vi "sumLinesIntoProjections.vi"(6 "calc ff/fb":bool, 7 "tracking":bool, 8 "error in (no error)":errorcluster, 10 "volumes to assemble":T3[](array[typedef])) -> (0 "error out":errorcluster, 1 "lines inserted":i32, 2 "volumes to send":cluster{"volume info":T1, "buffers":T2}[](array[cluster]), 3 "ch sums":cluster{"ch0 sum":u32, "ch1 sum":u32})   [LabVIEW 2010]
uses:
  volume_with_lines.ctl
  volume_info.ctl
  line_info.ctl
  projection buffers.ctl
  get write location projection.vi
  sum line into array.vi
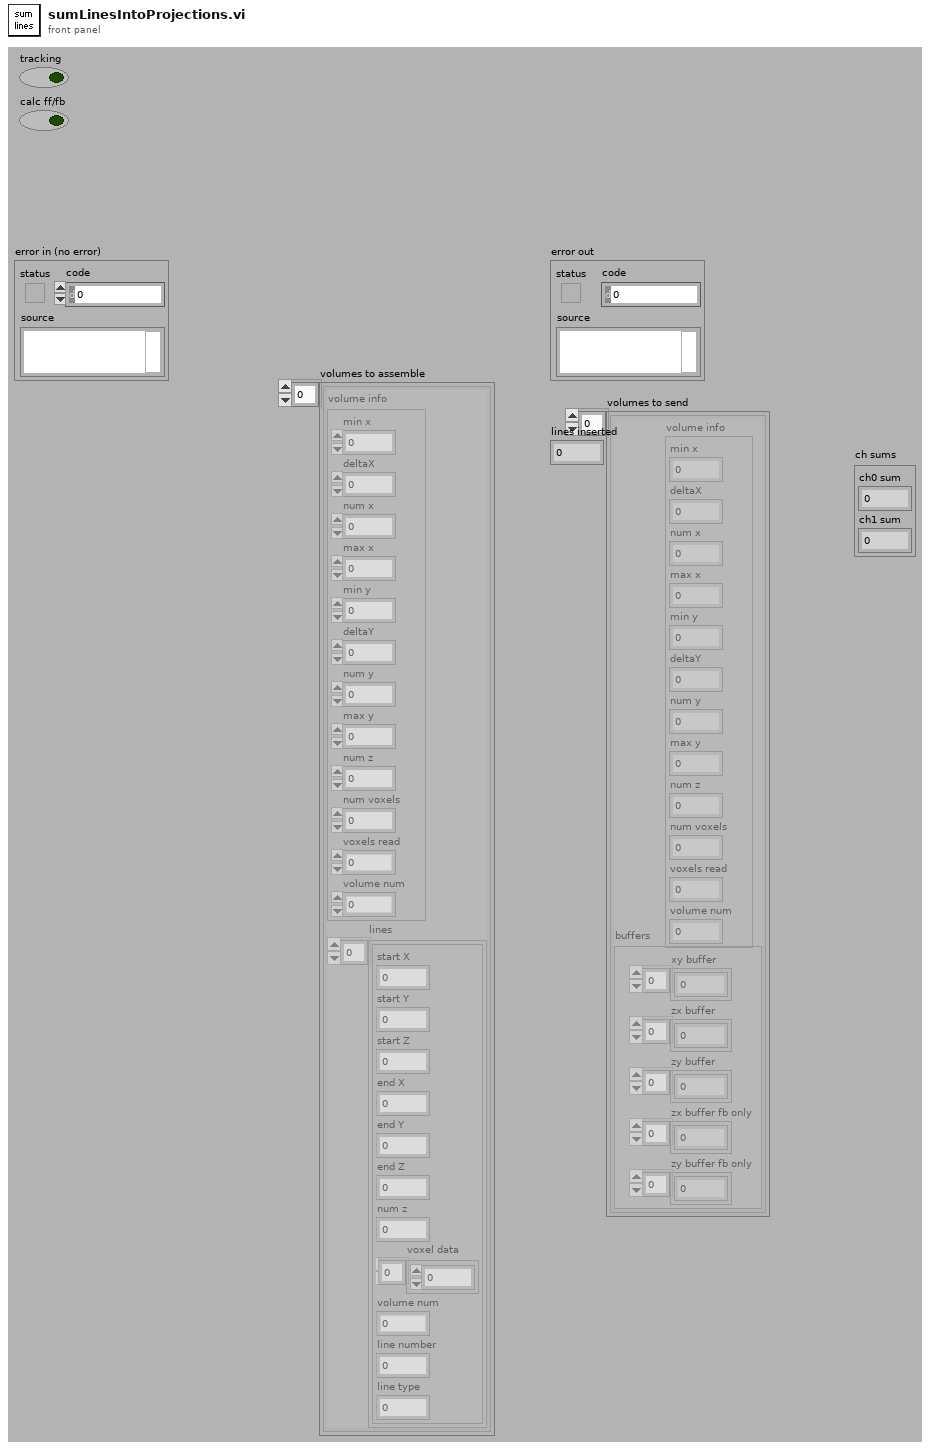
[diagram p1: front panel]
types:
  T1 = typedef "volume_info.ctl" = cluster{"min x":i16, "deltaX":dbl, "num x":u32, "max x":i16, "min y":i16, "deltaY":dbl, "num y":u32, "max y":i16, "num z":u32, "num voxels":u32, "voxels read":u32, "volume num":u32}
  T2 = typedef "projection buffers.ctl" = cluster{"xy buffer":u32[], "zx buffer":u32[], "zy buffer":u32[], "zx buffer fb only":u32[], "zy buffer fb only":u32[]}
  T3 = typedef "volume_with_lines.ctl" = cluster{"volume info":T1, "lines":T4[]}
  T4 = typedef "line_info.ctl" = cluster{"start X":i16, "start Y":i16, "start Z":i16, "end X":i16, "end Y":i16, "end Z":i16, "num z":u8, "voxel data":u32[], "volume num":u32, "line number":u16, "line type":u16}
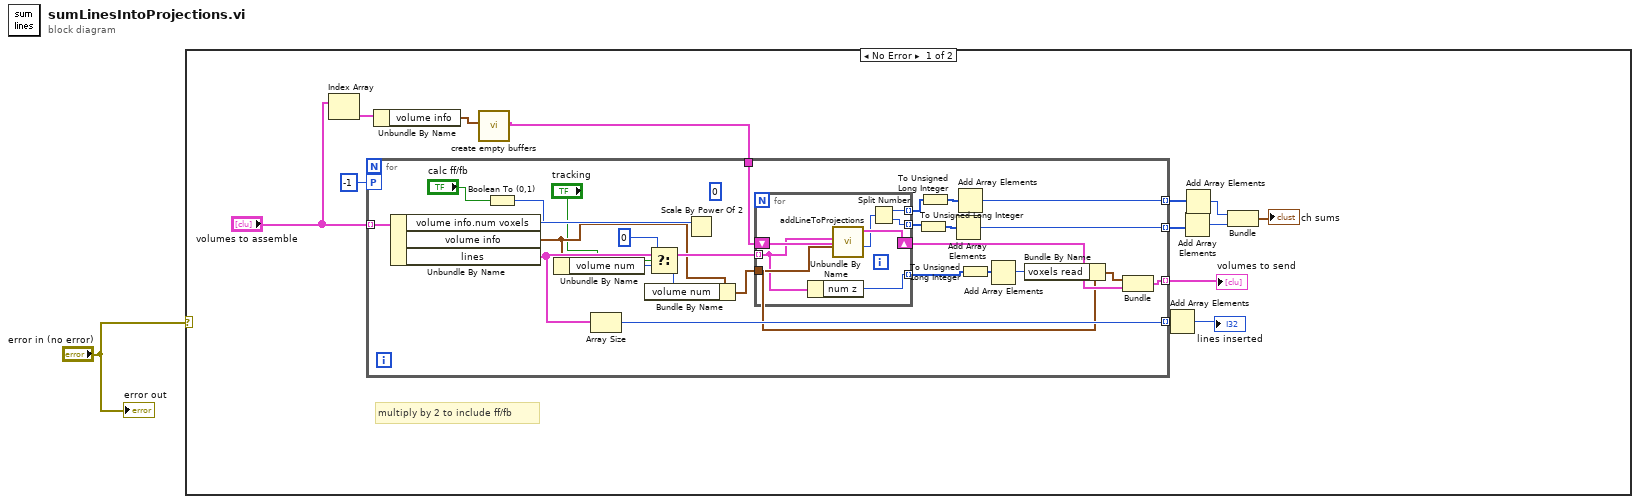
[diagram p0: block diagram]
diagram:
  n1 = case shown="No Error" "error in (no error)" {
    frame No Error {
      # "multiply by 2 to include ff/fb"
      n2 = Index Array(array="volumes to assemble") -> (element=w4:T3)  [unwired: 1 in]
      n3 = Unbundle By Name(w4) -> ("volume info"=w3:T1)
      n4 = call "create empty buffers.vi"("volume info"=w3) -> ("empty buffers"=w2:T2)  [unwired: 10 in]
      n5 = for {
        tunnel: "volumes to assemble" -> [w39] mode=indexing
        tunnel: [w33] -> w11 mode=indexing
        workers-P: -1 -> [_]
        tunnel: [w30] -> w13 mode=indexing
        tunnel: w2 -> [w21]
        tunnel: [w16] -> w10 mode=indexing
        tunnel: [w15] -> w9 mode=indexing
        (unwired) u32 0
        n6 = Unbundle By Name(w39) -> ("volume info.num voxels"=w38:u32, "volume info"=w27:T1, "lines"=w31:T4[])
        n7 = Boolean To (0,1)(Boolean="calc ff/fb") -> (0, 1=w29:i16)
        n8 = Unbundle By Name(w27) -> ("volume num"=w25:u32)
        n9 = Array Size(array=w31) -> (size(s)=w30:i32)
        n10 = Select(t=u32 0, s="tracking", f=w25) -> (s? t:f=w26:u32)
        n11 = Bundle By Name(cluster=w27, "volume num"=w26) -> (w22:T1)
        n12 = Scale By Power Of 2(n=w29, x=w38) -> ()  [unwired: 1 out]
        n13 = for {
          tunnel: w22 -> [w46]
          tunnel: w31 -> [w44] mode=indexing
          shift-right: [w43] -> w34
          shift-left: w21 -> [w45]
          tunnel: [w47] -> w37 mode=indexing
          tunnel: [w41] -> w20 mode=indexing
          tunnel: [w40] -> w17 mode=indexing
          n14 = Unbundle By Name(w44) -> ("num z"=w47:u8)
          n15 = call "addLineToProjections.vi"("current volume"=w46, "line"=w44, "buffers"=w45) -> ("line sum"=w42:u32, "buffers out"=w43:T2)  [unwired: 7 in]
          n16 = Split Number(x=w42) -> (hi(x)=w41:u16, lo(x)=w40:u16)
        }
        n17 = To Unsigned Long Integer(number=w17) -> (unsigned 32bit integer=w18:u32[])
        n18 = To Unsigned Long Integer(number=w20) -> (unsigned 32bit integer=w19:u32[])
        n19 = Add Array Elements(numeric array=w18) -> (sum=w15:u32)
        n20 = Add Array Elements(numeric array=w19) -> (sum=w16:u32)
        n21 = To Unsigned Long Integer(number=w37) -> (unsigned 32bit integer=w32:u32[])
        n22 = Add Array Elements(numeric array=w32) -> (sum=w36:u32)
        n23 = Bundle By Name(cluster=w22, "voxels read"=w36) -> (w35:T1)
        n24 = Bundle("volume info"=w35, "empty buffers"=w34) -> (w33:cluster{"volume info":T1, "empty buffers":T2})  [unwired: 1 in]
      }
      "volumes to send" <- w11
      n25 = Add Array Elements(numeric array=w13) -> (sum=→"lines inserted":i32)
      n26 = Add Array Elements(numeric array=w9) -> (sum=w8:u32)
      n27 = Add Array Elements(numeric array=w10) -> (sum=w7:u32)
      n28 = Bundle(w7, w8) -> (→"ch sums":cluster{u32, u32})  [unwired: 1 in]
    }
    frame Error {
    }
  }
  "error out" <- "error in (no error)"
